vi "Await.vi"(8 "error in (no error)":errorcluster, 10 "Timeout":i32=-1, 11 "Awaiter":refnum<k24>) -> (0 "error out":errorcluster, 2 "Timeout":bool, 3 "Awaiter":refnum<k24>)   [LabVIEW 2020, in "WebView2 Control.xctl"]
uses:
  WebView2 Control.xctl
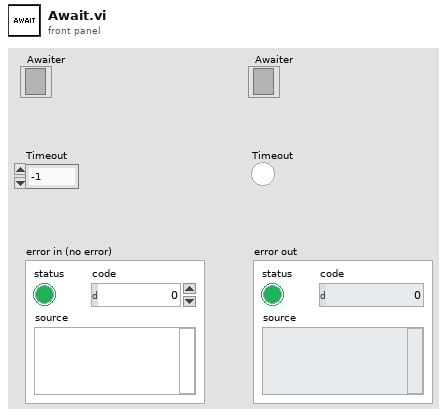
[diagram p1: front panel]
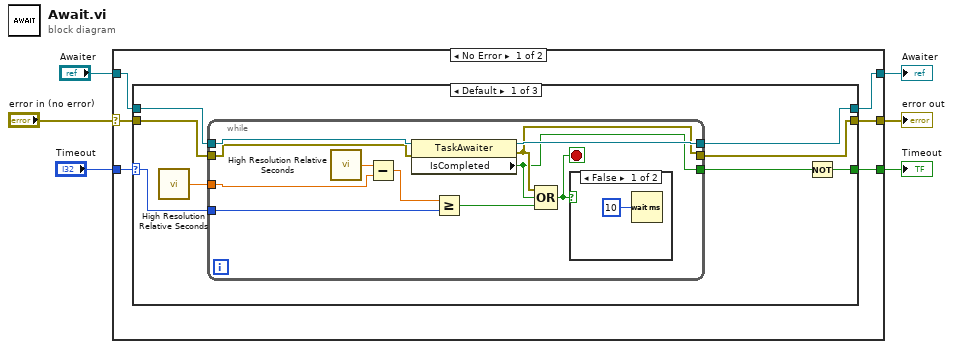
[diagram p0: block diagram]
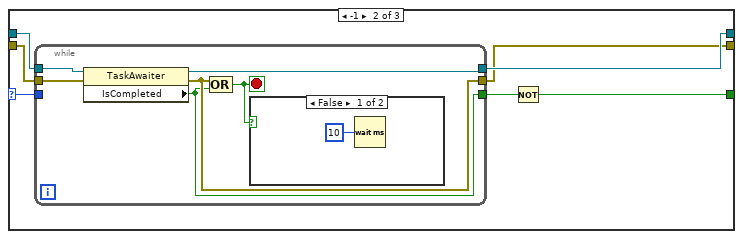
[diagram p3: hidden frame]
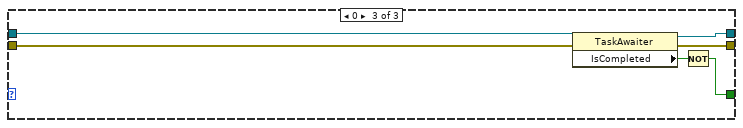
[diagram p5: hidden frame]
diagram:
  n1 = case shown="No Error" "error in (no error)" {
    selector: "error in (no error)" -> [w11 w54]
    tunnel: "Awaiter" -> [w12 w53]
    tunnel: [w10 w53] -> w4
    tunnel: "Timeout" -> [w9 _]
    tunnel: [w8 w54] -> w2
    tunnel: [w7 _] -> w1
    frame No Error {
      n2 = case shown="Default" w9 {
        selector: w9 -> [w17 w36 _]
        tunnel: w12 -> [w20 w39 w52]
        tunnel: w11 -> [w19 w38 w51]
        tunnel: [w18 w37 w50] -> w10
        tunnel: [w16 w35 w47] -> w8
        tunnel: [w13 w33 w48] -> w7
        frame Default {
          n3 = call <vilib>:"High Resolution Relative Seconds.vi"() -> ("relative seconds"=w15:dbl)
          n4 = while {
            tunnel: w20 -> [w31]
            tunnel: w19 -> [w30]
            tunnel: [w29] -> w18
            tunnel: w15 -> [w27]
            tunnel: w17 -> [w25]
            tunnel: [w23] -> w16
            tunnel: [w22] -> w14
            stop <- w21 stop-if-true
            n5 = call <vilib>:"High Resolution Relative Seconds.vi"() -> ("relative seconds"=w28:dbl)
            n6 = Subtract(x=w28, y=w27) -> (x-y=w26:dbl)
            n7 = property class="TaskAwaiter"(reference=w31, error in=w30) -> (reference out=w29:refnum<k24>, error out=w23:errorcluster, "IsCompleted"=w22:bool)
            n8 = Greater Or Equal?(x=w26, y=w25) -> (x >= y?=w24:bool)
            n9 = Compound Arithmetic op=OR(w23, w22, w24) -> (w21:bool)
            n10 = case shown="False" w21 {
              frame False {
                n11 = Wait (ms)(milliseconds to wait=u32 10) -> ()  [unwired: 1 out]
              }
              frame True {
              }
            }
          }
          n12 = Not(x=w14) -> (.not. x?=w13:bool)
        }
        frame -1 {
          n13 = while {
            tunnel: w39 -> [w45]
            tunnel: w38 -> [w44]
            tunnel: [w43] -> w37
            tunnel: w36 -> [_]
            tunnel: [w42] -> w35
            tunnel: [w41] -> w34
            stop <- w40 stop-if-true
            n14 = property class="TaskAwaiter"(reference=w45, error in=w44) -> (reference out=w43:refnum<k24>, error out=w42:errorcluster, "IsCompleted"=w41:bool)
            n15 = Compound Arithmetic op=OR(w42, w41) -> (w40:bool)
            n16 = case shown="False" w40 {
              frame False {
                n17 = Wait (ms)(milliseconds to wait=u32 10) -> ()  [unwired: 1 out]
              }
              frame True {
              }
            }
          }
          n18 = Not(x=w34) -> (.not. x?=w33:bool)
        }
        frame 0 {
          n19 = property class="TaskAwaiter"(reference=w52, error in=w51) -> (reference out=w50:refnum<k24>, error out=w47:errorcluster, "IsCompleted"=w49:bool)
          n20 = Not(x=w49) -> (.not. x?=w48:bool)
        }
      }
    }
    frame Error {
    }
  }
  "error out" <- w2
  "Timeout" <- w1
  "Awaiter" <- w4
